vi "Disconnect.vi"(8 "error in (no error)":errorcluster, 11 "GEN40-38-LAN in":refnum<class "GEN40-38-LAN.lvclass">) -> (0 "error out":errorcluster, 3 "GEN40-38-LAN out":refnum<class "GEN40-38-LAN.lvclass">)   [LabVIEW 2018, in "GEN40-38-LAN.lvlib" / "GEN40-38-LAN.lvclass"]
uses:
  GEN40-38-LAN.lvclass
  PPLs/Power Supply/Parent/Power_Supply.lvlibp/Power Supply.lvclass
  C:/Projects/LabVIEW/PPLs/Power Supply/Parent/Power_Supply.lvlibp/Power Supply.lvclass
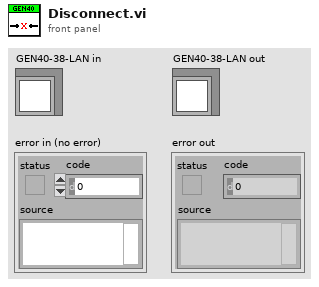
[diagram p1: front panel]
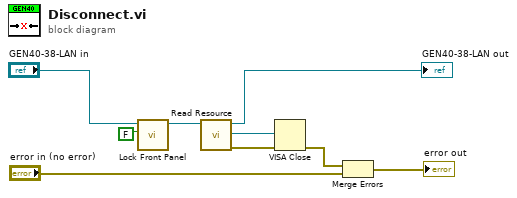
[diagram p0: block diagram]
diagram:
  n1 = call-dynamic "Lock Front Panel.vi"("Lock?"=FALSE, "GEN40-38-LAN in"="GEN40-38-LAN in") -> ("GEN40-38-LAN out"=w2:refnum<class "GEN40-38-LAN.lvclass">)  [unwired: 8 in, 1 out]
  n2 = call "Read Resource.vi"("Power Supply in"=w2) -> ("error out"=w8:errorcluster, "Resource"=w7:refnum<visa-resource-name>, "Power Supply out"=→"GEN40-38-LAN out":refnum<class "GEN40-38-LAN.lvclass">)  [unwired: 8 in]
  n3 = VISA Close(VISA resource name=w7, error in (no error)=w8) -> (error out=w6:errorcluster)
  n4 = Merge Errors(w6, "error in (no error)") -> (→"error out":errorcluster)
